vi "ThreePhasePLL_dev.vi"() -> ()   [LabVIEW 2017]
uses:
  <vilib>/Platform/TimedLoop/XDataNode/timing_clust.ctl
  <vilib>/Platform/TimedLoop/XDataNode/nitl_modes.ctl
  <vilib>/Platform/TimedLoop/XDataNode/wakeup.ctl
  <instrlib>/_niInstr/FIFO Register Bus/v1/FPGA/niInstr FIFO Register Bus v1 FPGA.lvclass
  C:/Program Files (x86)/National Instruments/LabVIEW 2017/instr.lib/_niInstr/Instruction Framework/v1/FPGA/Interfaces/Instruction Producer/Instruction Producer.lvclass
  <instrlib>/_niInstr/Instruction Framework/v1/FPGA/Helper Classes/Single Address Space Collection/Single Address Space Collection.lvclass
  C:/Program Files (x86)/National Instruments/LabVIEW 2017/instr.lib/_niInstr/Instruction Framework/v1/FPGA/Interfaces/Address Space Collection/Address Space Collection.lvclass
  <vilib>/rvi/Emulation/niFpgaGetClockAttributes.vi
  <vilib>/rvi/Emulation/niFpgaSctlEmulationGetInTimedLoop.vi
  <vilib>/rvi/Emulation/niFpgaEmulationReportErrorSimple.vi
  <userlib>/_NI FLP Library/FPGA/outsideSCTL/FlpLib Multiply Shared Instance 2.vi
  <userlib>/_NI FLP Library/FPGA/outsideSCTL/FlpLib Add Shared Instance 2.vi
  <userlib>/_NI FLP Library/FPGA/outsideSCTL/FlpLib Subtract Shared Instance 2.vi
  <userlib>/_NI FLP Library/FPGA/outsideSCTL/FlpLib Greater Than Shared Instance 2.vi
  <vilib>/rvi/Emulation/niFpgaProcessEmulError.vi
  <userlib>/_NI FLP Library/FPGA/outsideSCTL/FlpLib Cosine Shared Instance 2.vi
  <vilib>/rvi/Emulation/niFpgaCriticalErrorInLSC.vi
  <userlib>/_NI FLP Library/addons/PowerElectronics/ABCtoAlphaBeta_3PhaseUnitaryMagnitude/FlpLib ABCtoAlphaBeta_3PhaseUnitaryMagnitude 0.vi
  <userlib>/_NI FLP Library/FPGA/outsideSCTL/FlpLib Sine & Cosine Shared Instance 0.vi
  <userlib>/_NI FLP Library/addons/PowerElectronics/AlphaBetaToDQ_noSine/FlpLib AlphaBetaToDQ_noSine 0.vi
  <vilib>/rvi/interface/RandomDataEmulation/niFpgaRandomDataHandleErrors.vi
  <vilib>/rvi/DataTransferAndStorage/Container/XNode/niFpgaContainer.xnode
  <vilib>/rvi/interface/RandomDataEmulation/nirviRandomDataFpgaReadWriteTemplate.vi
  <vilib>/Platform/TimedLoop/XDataNode/XDataNode.xnode
  ThreePhasePLL.lvlib
  <instrlib>/_niInstr/Instruction Framework/v1/FPGA/Top Level Bus/Register Configuration/Register Configuration.lvclass
  <vilib>/Platform/TimedLoop/XDataNode/XDNodeRunTimeDep.lvlib
  AddressSpace.lvclass
panel:
  out "Locked":bool
  in  "HarmonicGain":sgl=100.0
  in  "HarmonicFreqRadPerSec":sgl=376.991 format="%#_13g"
  in  "fifo reg bus ctrl 0":u32
  out "fifo reg bus status 0":u32
  out "fifo reg bus data 0":u64
  in  "gain":sgl=100.0
  out "theta error":sgl
  out "freq error":sgl
  out "gridFrequency":sgl
  out "PLLTimingActual":u32
  in  "PLL_Timing":u32=400
  out "C":sgl
  out "B":sgl
  out "A":sgl
  out "gridTheta":sgl
  in  "GenFreqRadPerSec":sgl=376.991 format="%#_13g"
  in  "dTGen":sgl=1e-05 format="%#_13g"
  out "ThreePhaseGenActual":u32
  in  "ThreePhaseGenTiming":u32=400
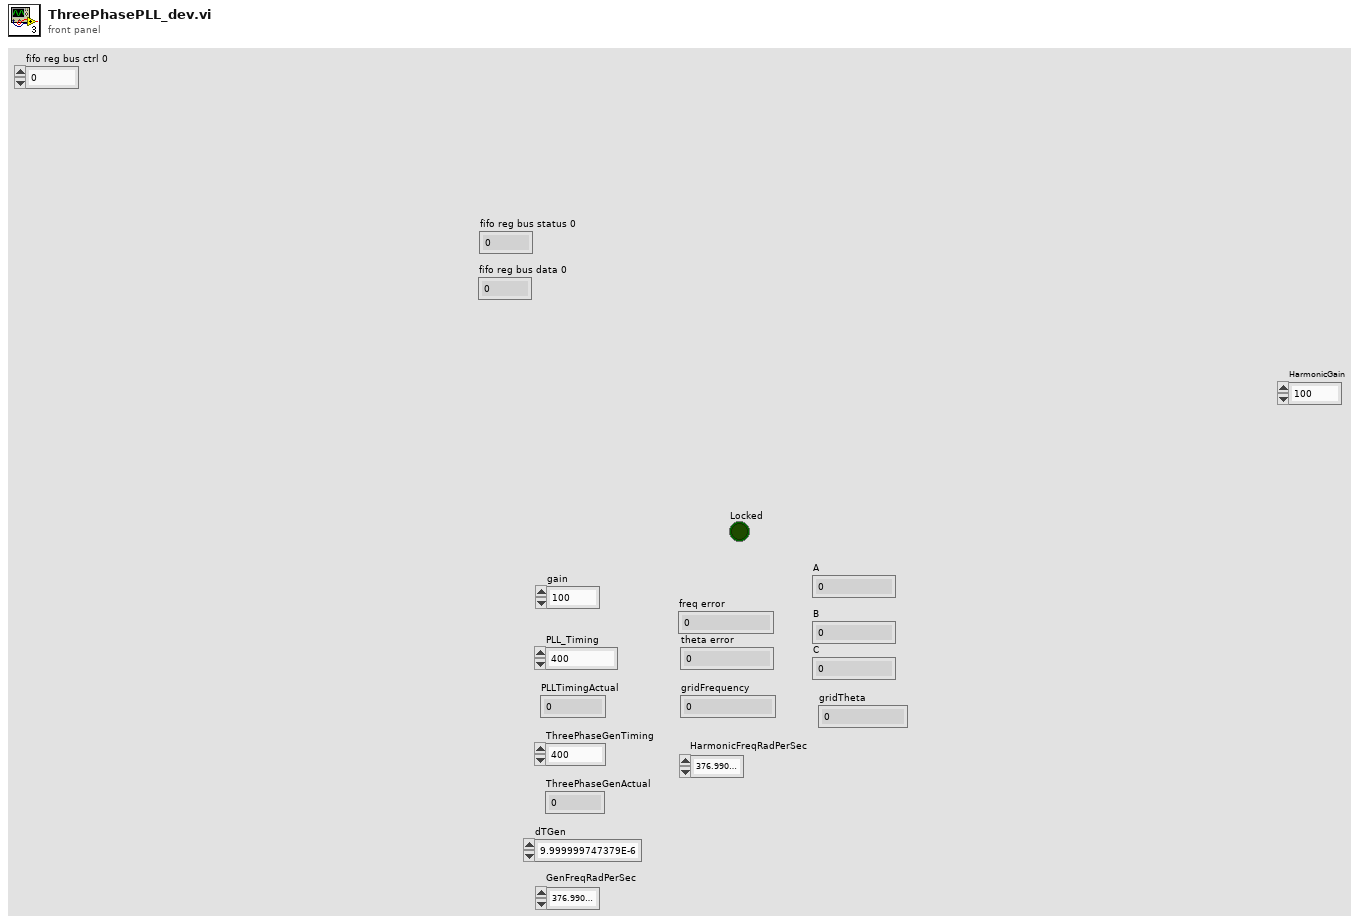
[diagram p1: front panel]
types:
  T1 = typedef "ThreePhasePLL.lvlib/registers.ctl" = cluster{"PLLGains":refnum<k21>, "PLLRange":refnum<k21>, "PLL_reset":refnum<k21>, "PLL_locked":refnum<k21>, "freqBoundaries":refnum<k21>, "expectedFreq":refnum<k21>, "lockDuration":refnum<k21>, "dT":refnum<k21>, "detectedFreq":refnum<k21>, "adjustTheta":refnum<k21>, "HarmonicFilter":refnum<k21>, "HarmonicFilterEnable":refnum<k21>}
  T2 = typedef "XDNodeRunTimeDep.lvlib/timing_clust.ctl" = cluster{"Expected End [f-1]":u64, "Actual End [f-1]":u64, "Finished Late? [f-1]":bool, "Expected End [i-1]":u64, "Actual End [i-1]":u64, "Finished Late? [i-1]":bool, "Expected Start [i]":u64, "Actual Start [i]":u64, "Expected Start [f]":u64, "Actual Start [f]":u64, "Source Name":string, "Structure Name":string, "Period":i64, "Deadline":i64, "Offset":i64, "Start":i64, "Priority":i32, "Timeout":i32, "Mode":T3, "Wakeup Reason":T4, "Error":errorcluster, "Source Type":string, "Secondary Source Type":string, "Global End Time":u64, "Global Start Time":u64, "Frame Duration":u64, "Iteration Duration":u64, "Assigned CPU":i32, "I/O Scan Engine Mode":u32}
  T3 = typedef "XDNodeRunTimeDep.lvlib/nitl_modes.ctl" = enum32{"No Change", "Process missed periods, maintain original phase", "Discard missed periods, maintain original phase", "Process missed periods, ignore original phase", "Discard missed periods, ignore original phase"}
  T4 = typedef "XDNodeRunTimeDep.lvlib/wakeup.ctl" = enum32{"Normal", "Aborted", "Asynchronous wakeup", "Timing source error", "Timed loop error", "Timeout"}
  T5 = typedef "niFpgaPID_PIState.ctl" = cluster{"uI(k-1)":sgl, "e(k-1)":sgl, "output (k-1)":sgl}
  T6 = cluster{"PIstateOut":T5, "filter0":sgl, "filter1":sgl}
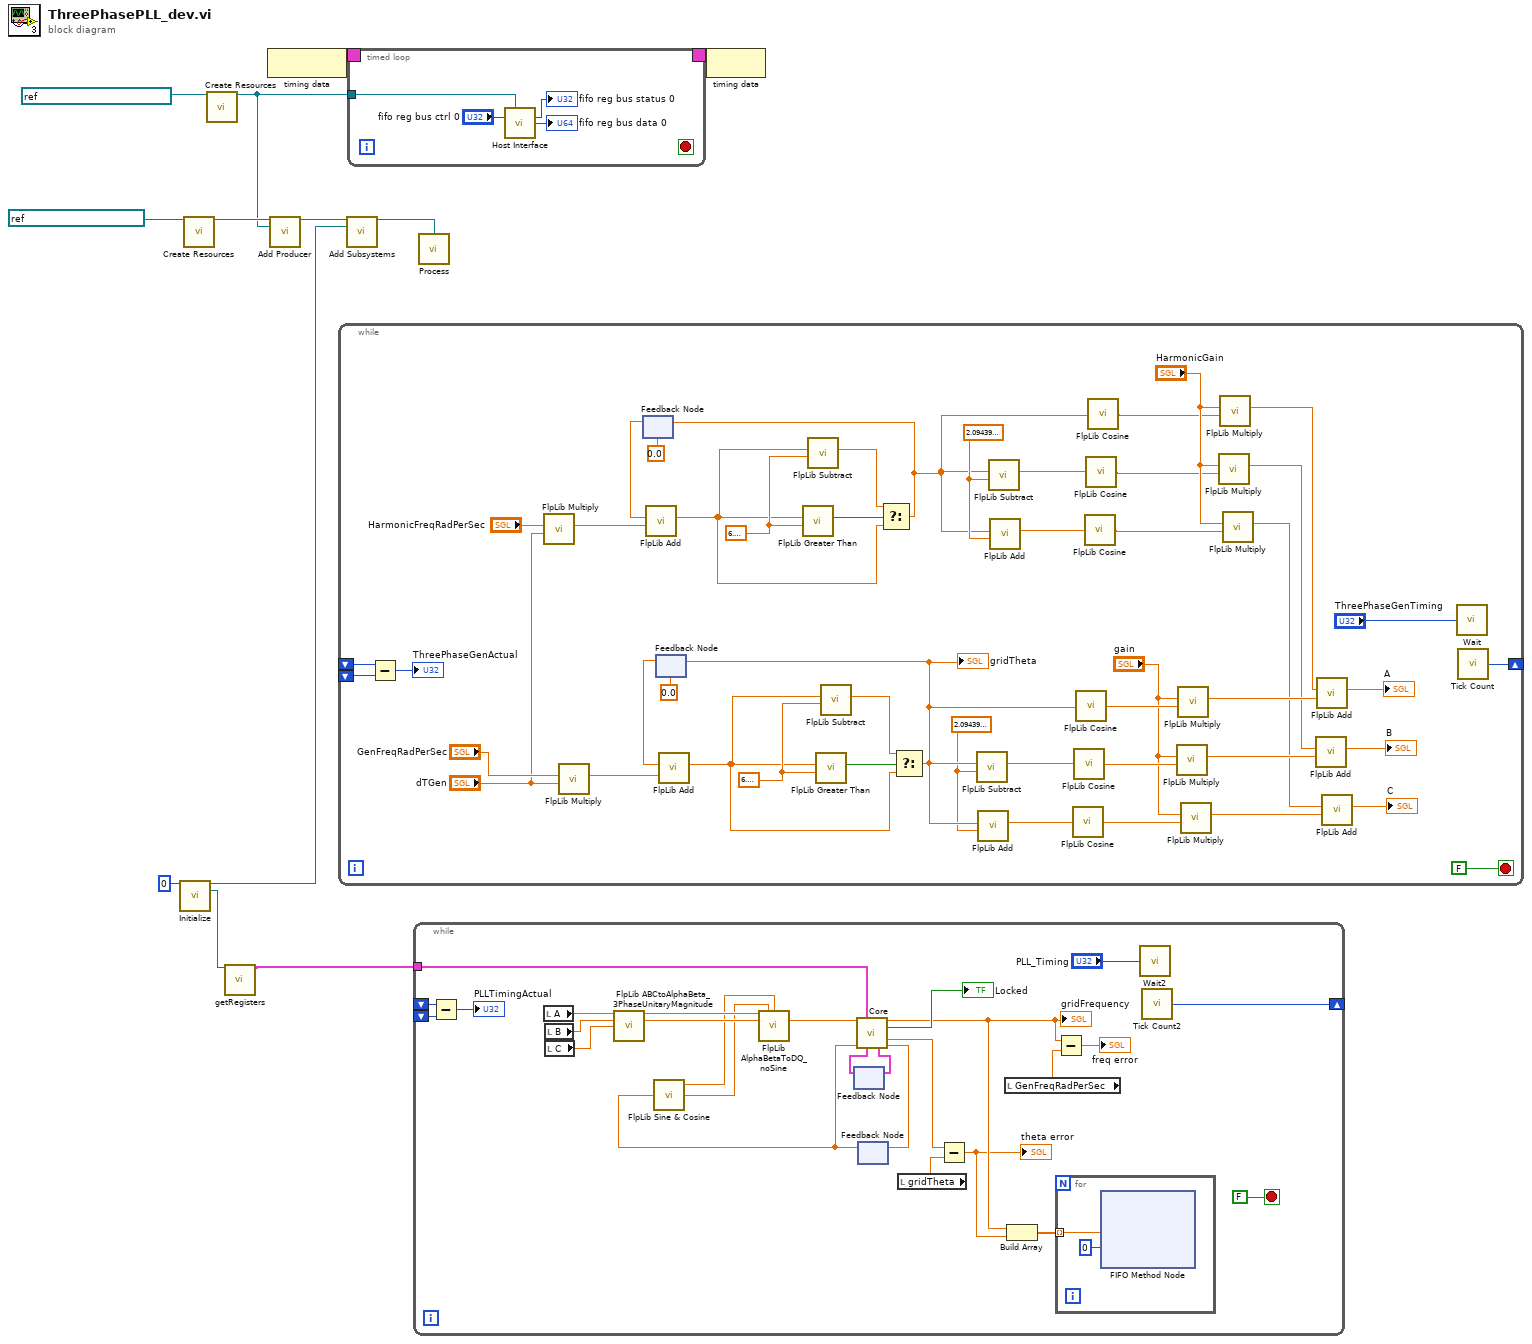
[diagram p0: block diagram]
diagram:
  n1 = call "Initialize.vi"("instance"=u8 0) -> ("subsysytem"=w2:refnum<class "Single Address Space Collection.lvclass">, "AddressSpace"=w4:refnum<class "AddressSpace.lvclass">)  [unwired: 13 in]
  n2 = call <instrlib>:"Create Resources.vi"("register clock"=refnum<k21> "40 MHz Onboard Clock") -> ("register configuration"=w8:refnum<class "Register Configuration.lvclass">)  [unwired: 14 in]
  n3 = call <instrlib>:"Create Resources.vi"("instruction fifo"=refnum<k21> "reg.host instruction fifo 0") -> ("fifo register bus"=w6:refnum<class "niInstr FIFO Register Bus v1 FPGA.lvclass">)  [unwired: 14 in]
  n4 = call "getRegisters.vi"("AddressSpace"=w4) -> ("registers"=w3:T1)  [unwired: 14 in]
  n5 = node-c288() -> (w12:T2)
  n6 = call <instrlib>:"Add Producer.vi"("register configuration in"=w8, "instruction producer"=w6) -> ("register configuration out"=w7:refnum<class "Register Configuration.lvclass">)  [unwired: 13 in]
  n7 = while {
    shift-right: [w59] -> _
    shift-left: _ -> [w44]
    shift-left: _ -> [w43]
    stop <- FALSE stop-if-true
    w28 = sgl 2.0944 ("y")
    w33 = sgl 6.2831855
    w47 = sgl 2.0944 ("y")
    w52 = sgl 6.2831855
    n8 = Subtract(x=w44, y=w43) -> (x-y=→"ThreePhaseGenActual":u32)
    n9 = call-poly <userlib>:"FlpLib Multiply.vi"("y"="dTGen", "x"="HarmonicFreqRadPerSec") -> ("x*y"=w30:sgl)  [unwired: 5 in]
    n10 = call-poly <userlib>:"FlpLib Multiply.vi"("y"="dTGen", "x"="GenFreqRadPerSec") -> ("x*y"=w54:sgl)  [unwired: 5 in]
    n11 = feedback #1(sgl 0.0) -> (w35:sgl)
    n12 = call-poly <userlib>:"FlpLib Add.vi"("y"=w30, "x"=w35) -> ("x+y"=w31:sgl)  [unwired: 5 in]
    n13 = feedback #2(sgl 0.0) -> (w55:sgl)
    n14 = call-poly <userlib>:"FlpLib Add.vi"("y"=w54, "x"=w55) -> ("x+y"=w50:sgl)  [unwired: 5 in]
    n15 = call-poly <userlib>:"FlpLib Greater Than.vi"("y"=w33, "x"=w31) -> ("x > y?"=w34:bool)  [unwired: 5 in]
    n16 = call-poly <userlib>:"FlpLib Subtract.vi"("y"=w33, "x"=w31) -> ("x-y"=w32:sgl)  [unwired: 5 in]
    n17 = call-poly <userlib>:"FlpLib Greater Than.vi"("y"=w52, "x"=w50) -> ("x > y?"=w53:bool)  [unwired: 5 in]
    n18 = call-poly <userlib>:"FlpLib Subtract.vi"("y"=w52, "x"=w50) -> ("x-y"=w51:sgl)  [unwired: 5 in]
    n19 = Select(t=w32, s=w34, f=w31) -> (s? t:f=w26:sgl)
    n20 = feedback-in #1(w26) -> ()
    n21 = Select(t=w51, s=w53, f=w50) -> (s? t:f=w48:sgl)
    "gridTheta" <- w48
    n22 = feedback-in #2(w48) -> ()
    n23 = call-poly <userlib>:"FlpLib Subtract.vi"("y"=w47, "x"=w48) -> ("x-y"=w49:sgl)  [unwired: 5 in]
    n24 = call-poly <userlib>:"FlpLib Add.vi"("y"=w47, "x"=w48) -> ("x+y"=w46:sgl)  [unwired: 5 in]
    n25 = call-poly <userlib>:"FlpLib Subtract.vi"("y"=w28, "x"=w26) -> ("x-y"=w29:sgl)  [unwired: 5 in]
    n26 = call-poly <userlib>:"FlpLib Add.vi"("y"=w28, "x"=w26) -> ("x+y"=w27:sgl)  [unwired: 5 in]
    n27 = call-poly <userlib>:"FlpLib Cosine.vi"("x"=w46) -> ("cos(x)"=w42:sgl)  [unwired: 4 in]
    n28 = call-poly <userlib>:"FlpLib Cosine.vi"("x"=w49) -> ("cos(x)"=w41:sgl)  [unwired: 4 in]
    n29 = call-poly <userlib>:"FlpLib Cosine.vi"("x"=w48) -> ("cos(x)"=w40:sgl)  [unwired: 4 in]
    n30 = call-poly <userlib>:"FlpLib Cosine.vi"("x"=w27) -> ("cos(x)"=w22:sgl)  [unwired: 4 in]
    n31 = call-poly <userlib>:"FlpLib Cosine.vi"("x"=w29) -> ("cos(x)"=w23:sgl)  [unwired: 4 in]
    n32 = call-poly <userlib>:"FlpLib Cosine.vi"("x"=w26) -> ("cos(x)"=w24:sgl)  [unwired: 4 in]
    n33 = call-poly <userlib>:"FlpLib Multiply.vi"("y"=w41, "x"="gain") -> ("x*y"=w18:sgl)  [unwired: 5 in]
    n34 = call-poly <userlib>:"FlpLib Multiply.vi"("y"=w40, "x"="gain") -> ("x*y"=w21:sgl)  [unwired: 5 in]
    n35 = call-poly <userlib>:"FlpLib Multiply.vi"("y"=w42, "x"="gain") -> ("x*y"=w15:sgl)  [unwired: 5 in]
    n36 = call-poly <userlib>:"FlpLib Multiply.vi"("y"=w23, "x"="HarmonicGain") -> ("x*y"=w16:sgl)  [unwired: 5 in]
    n37 = call-poly <userlib>:"FlpLib Multiply.vi"("y"=w24, "x"="HarmonicGain") -> ("x*y"=w20:sgl)  [unwired: 5 in]
    n38 = call-poly <userlib>:"FlpLib Multiply.vi"("y"=w22, "x"="HarmonicGain") -> ("x*y"=w13:sgl)  [unwired: 5 in]
    n39 = call-poly <userlib>:"FlpLib Add.vi"("y"=w18, "x"=w16) -> ("x+y"=→"B":sgl)  [unwired: 5 in]
    n40 = call-poly <userlib>:"FlpLib Add.vi"("y"=w21, "x"=w20) -> ("x+y"=→"A":sgl)  [unwired: 5 in]
    n41 = call-poly <userlib>:"FlpLib Add.vi"("y"=w15, "x"=w13) -> ("x+y"=→"C":sgl)  [unwired: 5 in]
    n42 = call "Wait"("Count(Ticks)"="ThreePhaseGenTiming") -> ()  [unwired: 1 out]
    n43 = call "Tick Count"() -> ("Tick Count(Ticks)"=w59:u32)
  }
  n44 = call <instrlib>:"Add Subsystems.vi"("register configuration in"=w7, "subsystems"=w2) -> ("register configuration out"=w5:refnum<class "Register Configuration.lvclass">)  [unwired: 13 in]
  n45 = timed-loop {
    timing: w12 -> [_]
    timing-out: [_] -> w11
    tunnel: w6 -> [w64]
    stop <- _ stop-if-true
    n46 = call <instrlib>:"Host Interface.vi"("fifo register bus"=w64, "fifo reg bus ctrl 0"="fifo reg bus ctrl 0") -> ("fifo reg bus status 0"=→"fifo reg bus status 0":u32, "fifo reg bus data 0"=→"fifo reg bus data 0":u64)  [unwired: 12 in]
  }
  n47 = while {
    shift-right: [w87] -> _
    shift-left: _ -> [w86]
    shift-left: _ -> [w85]
    tunnel: w3 -> [w74]
    stop <- FALSE stop-if-true
    n48 = Subtract(x=w86, y=w85) -> (x-y=→"PLLTimingActual":u32)
    n49 = local read "A"() -> (w93:sgl)
    n50 = local read "B"() -> (w92:sgl)
    n51 = local read "C"() -> (w91:sgl)
    n52 = call-poly <userlib>:"FlpLib ABCtoAlphaBeta_3PhaseUnitaryMagnitude.vi"("A"=w93, "B"=w92, "C"=w91) -> ("alpha"=w90:sgl, "beta"=w89:sgl)  [unwired: 11 in]
    n53 = feedback #3() -> (w71:T6)  [unwired: 1 in]
    n54 = feedback #4() -> (w75:sgl)  [unwired: 1 in]
    n55 = call-poly <userlib>:"FlpLib Sine & Cosine.vi"("x"=w75) -> ("cos(x)"=w82:sgl, "sin(x)"=w81:sgl)  [unwired: 3 in]
    n56 = call-poly <userlib>:"FlpLib AlphaBetaToDQ_noSine.vi"("alpha"=w90, "cosx"=w82, "sinx"=w81, "beta"=w89) -> ("quadrature"=w77:sgl)  [unwired: 10 in, 1 out]
    n57 = call "Core.vi"("Vq"=w77, "registers"=w74, "ThetaIn"=w75, "StateIn"=w71) -> ("gridFrequency"=w69:sgl, "Locked"=→"Locked":bool, "adjustedTheta"=w73:sgl, "StateOut"=w72:T6, "ThetaOut"=w76:sgl)  [unwired: 7 in]
    "gridFrequency" <- w69
    n58 = feedback-in #3(w72) -> ()
    n59 = feedback-in #4(w76) -> ()
    n60 = local read "gridTheta"() -> (w78:sgl)
    n61 = Subtract(x=w73, y=w78) -> (x-y=w68:sgl)
    "theta error" <- w68
    n62 = local read "GenFreqRadPerSec"() -> (w80:sgl)
    n63 = Build Array(w69, w68) -> (w67:sgl[])
    n64 = Subtract(x=w69, y=w80) -> (x-y=→"freq error":sgl)
    n65 = for {
      tunnel: w67 -> [w95] mode=indexing
      n66 = xnode ("FIFO Method Node")("Element"=w95, "Timeout"=0) -> ()  [unwired: 1 in, 2 out]
    }
    n67 = call "Wait2"("Count(Ticks)"="PLL_Timing") -> ()  [unwired: 1 out]
    n68 = call "Tick Count2"() -> ("Tick Count(Ticks)"=w87:u32)
  }
  n69 = call <instrlib>:"Process.vi"("register configuration"=w5) -> ()  [unwired: 15 in]
  n70 = node-c288(w11) -> ()
